vi "MidRight.vi"   [LabVIEW 2017]
types:
  T1 = typedef "Command Status Info.ctl" = cluster{"Name":string, "Status":T2, "notifier out":T3}
  T2 = typedef "Completion Status.ctl" = enum16{"Successful", "Aborted", "Incomplete"}
  T3 = typedef "Completion Notifier.ctl" = refnum<notifier>
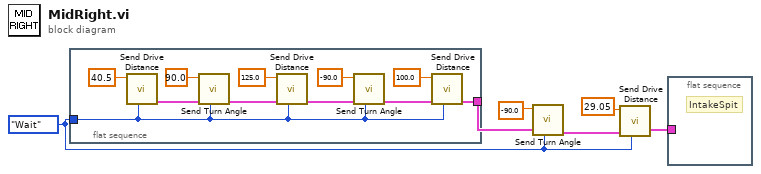
[diagram p0: block diagram]
diagram:
  w6 = enum16{"Start", "Wait"}."Wait" ("Synchronization")
  n1 = flat-sequence {
    tunnel: w6 -> [w8]
    tunnel: [w7] -> w2
    frame #0 {
      n2 = call "Send Drive Distance.vi"("Synchronization"=w8, "Target Distance"=40.5) -> ("Command Info Out"=w13:T1)  [unwired: 8 in, 1 out]
      n3 = call "Send Turn Angle.vi"("Synchronization"=w8, "Command Info In"=w13, "Target Angle"=90.0) -> ("Command Info Out"=w12:T1)  [unwired: 7 in, 1 out]
      n4 = call "Send Drive Distance.vi"("Synchronization"=w8, "Command Info In"=w12, "Target Distance"=125.0) -> ("Command Info Out"=w11:T1)  [unwired: 7 in, 1 out]
      n5 = call "Send Turn Angle.vi"("Synchronization"=w8, "Command Info In"=w11, "Target Angle"=-90.0) -> ("Command Info Out"=w10:T1)  [unwired: 7 in, 1 out]
      n6 = call "Send Drive Distance.vi"("Synchronization"=w8, "Command Info In"=w10, "Target Distance"=100.0) -> ("Command Info Out"=w7:T1)  [unwired: 7 in, 1 out]
    }
  }
  n7 = call "Send Turn Angle.vi"("Synchronization"=w6, "Command Info In"=w2, "Target Angle"=-90.0) -> ("Command Info Out"=w4:T1)  [unwired: 7 in, 1 out]
  n8 = call "Send Drive Distance.vi"("Synchronization"=w6, "Command Info In"=w4, "Target Distance"=29.05) -> ("Command Info Out"=w5:T1)  [unwired: 7 in, 1 out]
  n9 = flat-sequence {
    tunnel: w5 -> [_]
    frame #0 {
      # "IntakeSpit"
    }
  }
